vi "ConvertDateToJulianDay.vi"(11 "date in":string) -> (1 "strJulianDay":string, 2 "nJulianDay":i32, 3 "평년?":bool)   [LabVIEW 2018, in "Library-DataConvert.lvlib"]
uses:
  Library-DataConvert.lvlib
panel:
  # "20010916\nyyyymmdd"
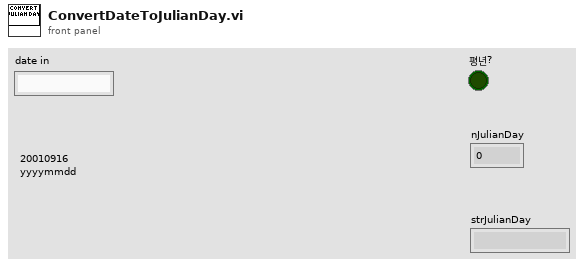
[diagram p1: front panel]
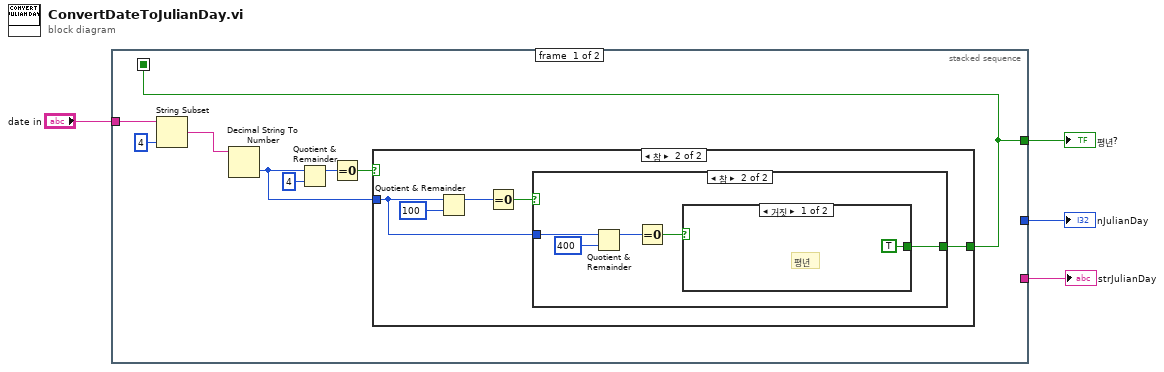
[diagram p0: block diagram]
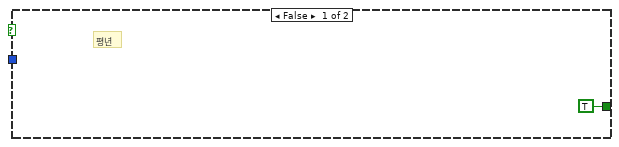
[diagram p2: hidden frame]
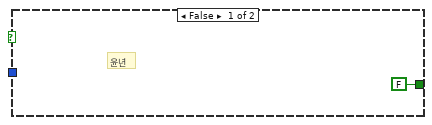
[diagram p3: hidden frame]
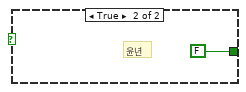
[diagram p4: hidden frame]
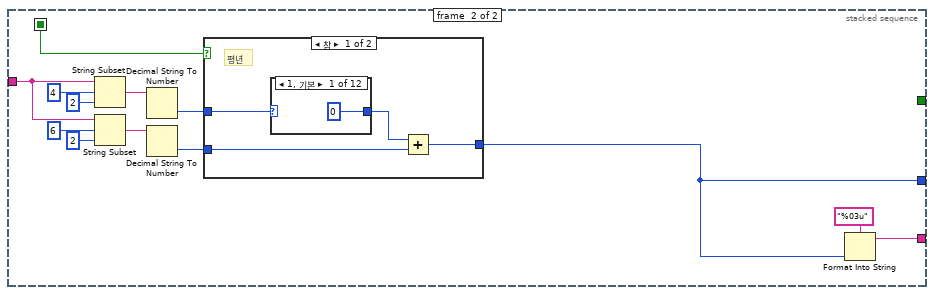
[diagram p5: hidden frame]
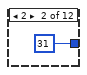
[diagram p6: hidden frame]
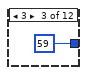
[diagram p7: hidden frame]
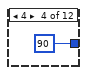
[diagram p8: hidden frame]
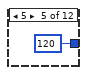
[diagram p9: hidden frame]
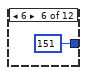
[diagram p10: hidden frame]
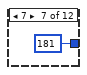
[diagram p11: hidden frame]
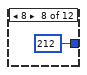
[diagram p12: hidden frame]
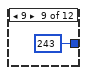
[diagram p13: hidden frame]
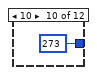
[diagram p14: hidden frame]
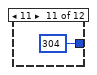
[diagram p15: hidden frame]
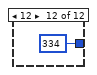
[diagram p16: hidden frame]
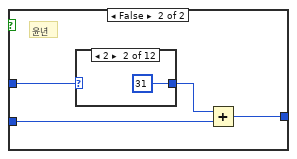
[diagram p17: hidden frame]
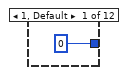
[diagram p18: hidden frame]
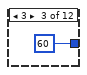
[diagram p19: hidden frame]
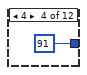
[diagram p20: hidden frame]
diagram:
  n1 = stacked-sequence {
    seq-local: [w5 _] -> [_ w34]
    tunnel: "date in" -> [w12 w35]
    tunnel: [w5 _] -> w3
    tunnel: [_ w28] -> w2
    tunnel: [_ w27] -> w1
    frame #0 {
      n2 = String Subset(string=w12, length (rest)=4 ("길이(나머지)")) -> (substring=w10:string)  [unwired: 1 in]
      n3 = Decimal String To Number(string=w10) -> (number=w6:i32)  [unwired: 2 in, 1 out]
      n4 = Quotient & Remainder(x=w6, y=4) -> (x-y*floor(x/y)=w8:i32)  [unwired: 1 out]
      n5 = Equal To 0?(x=w8) -> (x = 0?=w7:bool)
      n6 = case shown="참" w7 {
        tunnel: w6 -> [_ w15]
        tunnel: [TRUE w14] -> w5
        frame False {
          # "평년"
        }
        frame True {
          n7 = Quotient & Remainder(x=w15, y=100) -> (x-y*floor(x/y)=w17:i32)  [unwired: 1 out]
          n8 = Equal To 0?(x=w17) -> (x = 0?=w16:bool)
          n9 = case shown="참" w16 {
            tunnel: w15 -> [_ w23]
            tunnel: [FALSE w20] -> w14
            frame False {
              # "윤년"
            }
            frame True {
              n10 = Quotient & Remainder(x=w23, y=400) -> (x-y*floor(x/y)=w22:i32)  [unwired: 1 out]
              n11 = Equal To 0?(x=w22) -> (x = 0?=w21:bool)
              n12 = case shown="거짓" w21 {
                tunnel: [TRUE FALSE] -> w20
                frame False {
                  # "평년"
                }
                frame True {
                  # "윤년"
                }
              }
            }
          }
        }
      }
    }
    frame #1 {
      n13 = String Subset(string=w35, offset (0)=4 ("길이(나머지)"), length (rest)=2 ("길이(나머지)")) -> (substring=w33:string)
      n14 = String Subset(string=w35, offset (0)=6 ("길이(나머지)"), length (rest)=2 ("길이(나머지)")) -> (substring=w32:string)
      n15 = Decimal String To Number(string=w33) -> (number=w31:i32)  [unwired: 2 in, 1 out]
      n16 = Decimal String To Number(string=w32) -> (number=w30:i32)  [unwired: 2 in, 1 out]
      n17 = case shown="참" w34 {
        tunnel: w31 -> [w43 w59]
        tunnel: w30 -> [w42 w58]
        tunnel: [w40 w56] -> w28
        frame True {
          # "평년"
          n18 = case shown="1, 기본" w43 {
            tunnel: [0 31 59 90 120 151 181 212 243 273 304 334] -> w41
            frame 1, Default {
            }
            frame 2 {
            }
            frame 3 {
            }
            frame 4 {
            }
            frame 5 {
            }
            frame 6 {
            }
            frame 7 {
            }
            frame 8 {
            }
            frame 9 {
            }
            frame 10 {
            }
            frame 11 {
            }
            frame 12 {
            }
          }
          n19 = Add(x=w41, y=w42) -> (x+y=w40:i32)
        }
        frame False {
          # "윤년"
          n20 = case shown="2" w59 {
            tunnel: [0 31 60 91 121 152 182 213 244 274 305 335] -> w57
            frame 1, Default {
            }
            frame 2 {
            }
            frame 3 {
            }
            frame 4 {
            }
            frame 5 {
            }
            frame 6 {
            }
            frame 7 {
            }
            frame 8 {
            }
            frame 9 {
            }
            frame 10 {
            }
            frame 11 {
            }
            frame 12 {
            }
          }
          n21 = Add(x=w57, y=w58) -> (x+y=w56:i32)
        }
      }
      n22 = Format Into String(format string="%03u" ("포맷 문자열"), w28) -> (resulting string=w27:string)  [unwired: 2 in, 1 out]
    }
  }
  "평년?" <- w3
  "nJulianDay" <- w2
  "strJulianDay" <- w1
